vi "CheckLibraryInUse.vi"(8 "ErrorIn":errorcluster caption="Error In(no Error)", 9 "ErrorCode":i32, 10 "Library":string, 11 "ReferenceIn":refnum<class "ErrorDefinitionSQLite.lvclass"> caption="Reference In") -> (0 "ErrorOut":errorcluster caption="Error Out", 1 "LibraryInUse":bool, 2 "SpecificErrorInUse":bool, 3 "ReferenceOut":refnum<class "ErrorDefinitionSQLite.lvclass"> caption="Reference Out")   [LabVIEW 2021, in "ErrorDefinitionSQLite.lvclass"]
uses:
  ErrorDefinitionSQLite.lvclass
  <vilib>/drjdpowell/SQLite Library/SQL Connection/Execute SQL.vi
  <vilib>/drjdpowell/SQLite Library/SQLite.lvlib
  <vilib>/drjdpowell/SQLite Library/SQL Connection/Connection.lvclass
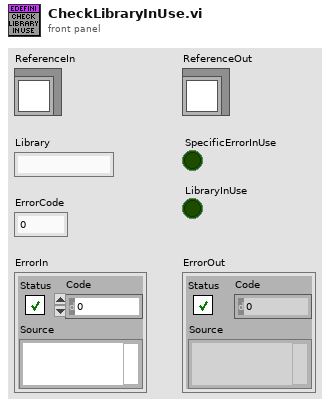
[diagram p1: front panel]
types:
  T1 = typedef "ErrorDefinitionSQLite.lvclass/ObjectAttributes.ctl" = cluster{"Path":path, "SQLiteRef":refnum<class "Connection.lvclass">, "EndOfRange":i32, "DefaultLibrarySize":i32, "StartOfRange":i32}
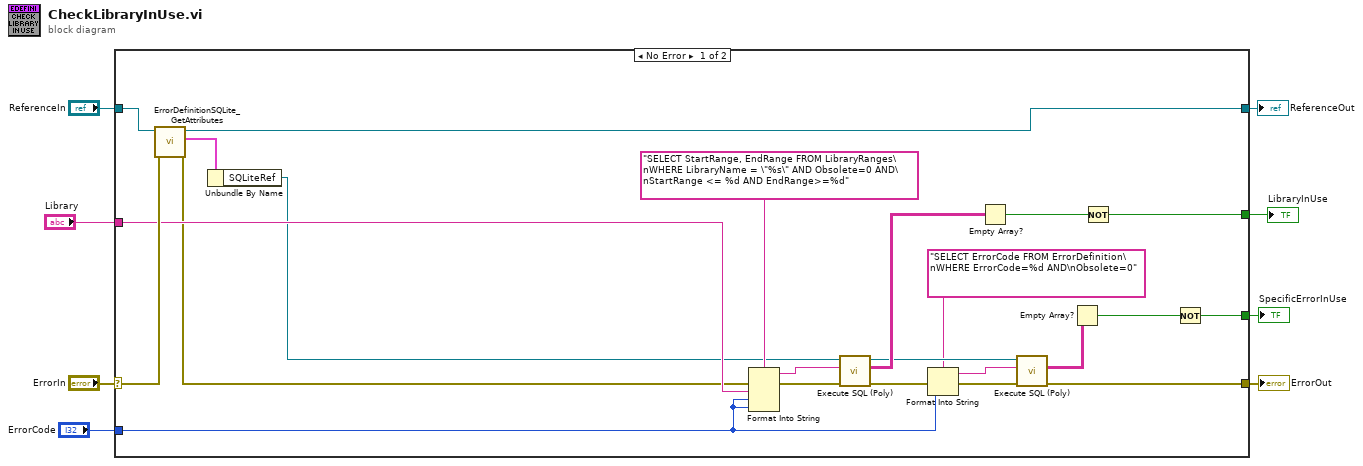
[diagram p0: block diagram]
diagram:
  n1 = case shown="No Error" "ErrorIn" {
    selector: "ErrorIn" -> [w31 w33]
    tunnel: [w19 w33] -> w7
    tunnel: [w29 w32] -> w5
    tunnel: "ReferenceIn" -> [w30 w32]
    tunnel: "ErrorCode" -> [w11 _]
    tunnel: "Library" -> [w24 _]
    tunnel: [w21 _] -> w2
    tunnel: [w15 _] -> w1
    frame No Error {
      n2 = call "ErrorDefinitionSQLite_GetAttributes.vi"("ErrorIn"=w31, "Reference in"=w30) -> ("ErrorOut"=w10:errorcluster, "Data"=w28:T1, "Reference out"=w29:refnum<class "ErrorDefinitionSQLite.lvclass">)  [unwired: 6 in, 1 out]
      n3 = Unbundle By Name(w28) -> ("SQLiteRef"=w9:refnum<class "Connection.lvclass">)
      n4 = Format Into String(format string="SELECT StartRange, EndRange FROM LibraryRanges\nWHERE LibraryName = \"%s\" AND Obsolete=0 AND\nStartRange <= %d AND EndRange>=%d" ("SQL"), error in=w10, w24, w11, w11) -> (resulting string=w27:string, error out=w26:errorcluster)  [unwired: 1 in]
      n5 = call-poly <vilib>:"Execute SQL (Poly).vi"("error in (no error)"=w26, "SQL"=w27, "SQLite Connection in"=w9) -> ("error out"=w20:errorcluster, "Result Set"=w23:string[][], "SQLite Connection"=w18:refnum<class "Connection.lvclass">)  [unwired: 5 in, 1 out]
      n6 = Format Into String(format string="SELECT ErrorCode FROM ErrorDefinition\nWHERE ErrorCode=%d AND\nObsolete=0" ("SQL"), error in=w20, w11) -> (resulting string=w12:string, error out=w14:errorcluster)  [unwired: 1 in]
      n7 = Empty Array?(array=w23) -> (empty?=w22:bool)
      n8 = call-poly <vilib>:"Execute SQL (Poly).vi"("error in (no error)"=w14, "SQL"=w12, "SQLite Connection in"=w18) -> ("error out"=w19:errorcluster, "Result Set"=w16:string[][])  [unwired: 5 in, 2 out]
      n9 = Empty Array?(array=w16) -> (empty?=w17:bool)
      n10 = Not(x=w22) -> (.not. x?=w21:bool)
      n11 = Not(x=w17) -> (.not. x?=w15:bool)
    }
    frame Error {
    }
  }
  "ErrorOut" <- w7
  "ReferenceOut" <- w5
  "LibraryInUse" <- w2
  "SpecificErrorInUse" <- w1
